vi "模态分析.vi"() -> ()   [LabVIEW 2014]
uses:
  <vilib>/Analysis/4window.llb/windowTd.ctl
  <vilib>/Utility/error.llb/DialogType.ctl
  <vilib>/Analysis/3filter.llb/Filter Structure Type.ctl
  <vilib>/DAQmx/read.llb/DAQmx Read (Analog 1D Wfm NChan NSamp).vi
  <vilib>/Analysis/2dsp.llb/Inverse Real FFT.vi
  <vilib>/DAQmx/create/channels.llb/DAQmx Create Channel (AI-Voltage-Basic).vi
  <vilib>/DAQmx/configure/timing.llb/DAQmx Timing (Sample Clock).vi
  <vilib>/DAQmx/miscellaneous.llb/DAQmx Fill In Error Info.vi
  <vilib>/measure/macond.llb/IIR Filter for 1 Chan.vi
  <vilib>/measure/maspectr.llb/Frequency Response Function (Mag-Phase) 1-1.vi
  <vilib>/measure/NI_MAPro.lvlib
  <vilib>/Analysis/NI_AALPro.lvlib
  <vilib>/Analysis/NI_AALBase.lvlib
panel:
  in  "units 2":i32(ring)=10348 caption="单位" items=["伏特"=10348, "来自自定义换算"=10065]
  in  "units":i32(ring)=10348 caption="单位" items=["伏特"=10348, "来自自定义换算"=10065]
  in  "触发阈值":dbl
  in  "Upper Fc":dbl
  in  "Lower Fc":dbl
  in  "Order":i32
  out "X":dbl[](array[numeric])
  in  "averaging mode":T1(ring)
  in  "是否转换成dB":bool=TRUE
  out "相关函数":cluster{"f0":dbl, "df":dbl, "coherence":dbl[]}(graph)
  out "相位":cluster{"f0":dbl, "df":dbl, "phase":dbl[]}(graph)
  out "幅度":cluster{"f0":dbl, "df":dbl, "magnitude":dbl[]}(graph)
  in  "FRF Mode":enum16{"H1", "H2", "H3"}(ring) caption="FRF模式"
  in  "window":T2=1 caption="窗" items=["矩形"=0, "Hanning"=1, "Hamming"=2, "Blackman-Harris"=3, "Exact Blackman"=4, "Blackman"=5, "Flat Top"=6, "4阶Blackman-Harris "=7, "7阶Blackman-Harris"=8, "Low Sidelobe"=9, "Blackman Nuttall"=11, "三角"=30, "Bartlett-Hanning"=31, "Bohman"=32, "Parzen"=33, "Welch"=34, "Kaiser"=60, "Dolph-Chebyshev"=61, "高斯"=62]
  out "响应信号":waveform(dbl)(graph)
  out "激振信号":waveform(dbl)(graph)
  in  "number of samples per channel 2":i32=-1 caption="每通道采样数"
  in  "sample mode 2":i32(ring)=10178 caption="采样模式" items=["有限采样"=10178, "连续采样"=10123, "硬件定时单点"=12522]
  in  "rate 2":dbl=1000.0 caption="速率" format="%0.2f"
  in  "input terminal configuration 3":i32(ring)=-1 caption="输入接线端配置" items=["默认"=-1, "RSE"=10083, "NRSE"=10078, "差分"=10106, "伪差分"=12529]
  in  "DAQmx物理通道 2":tag
  in  "input terminal configuration 2":i32(ring)=-1 caption="输入接线端配置" items=["默认"=-1, "RSE"=10083, "NRSE"=10078, "差分"=10106, "伪差分"=12529]
  in  "DAQmx物理通道":tag
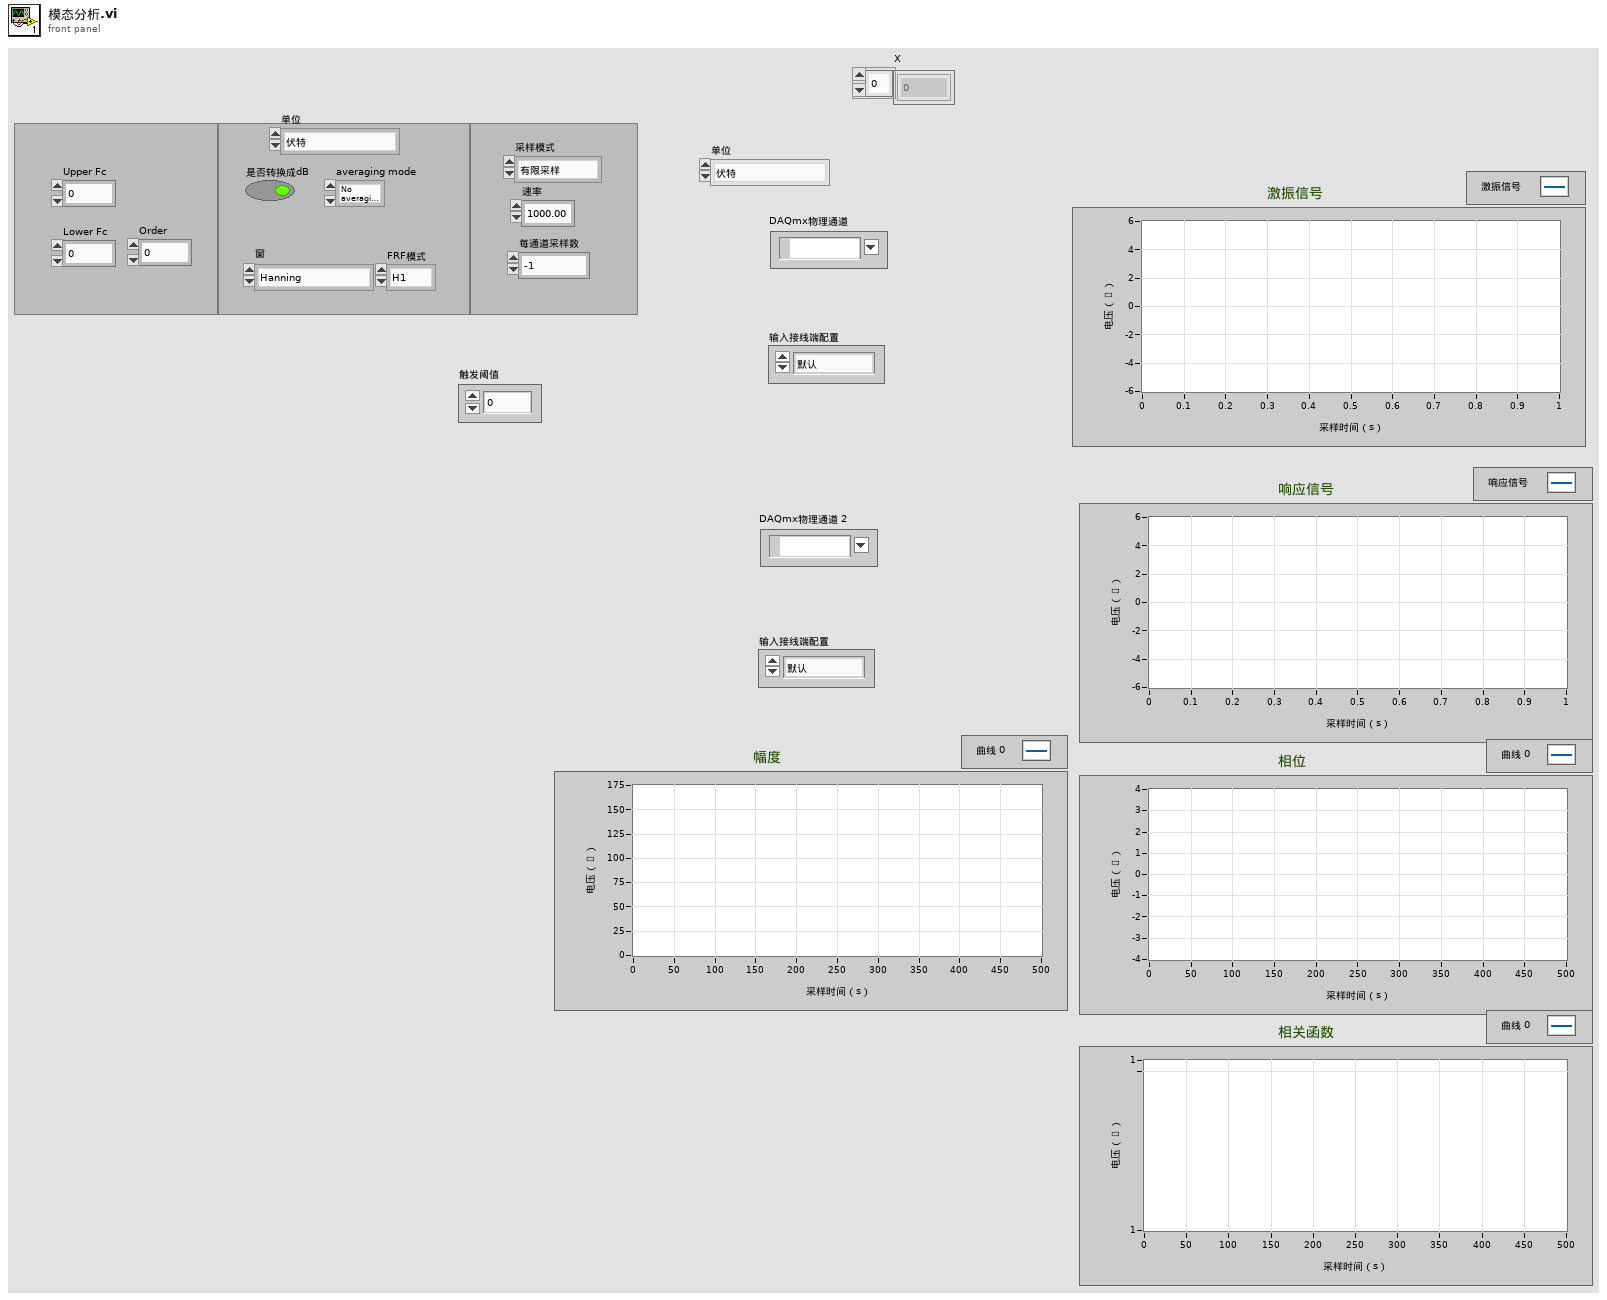
[diagram p1: front panel]
types:
  T1 = enum16{"No averaging", "Vector averaging", "RMS averaging", "Peak hold"}
  T2 = typedef "NI_AALPro.lvlib/windowTd.ctl" = u32
  T3 = typedef "NI_AALBase.lvlib/Filter Structure Type.ctl" = u16
  T4 = cluster{"Topology":enum16{"Off", "Butterworth", "Chebyshev", "Inverse Chebyshev", "Elliptic", "Bessel"}, "Type":enum16{"Lowpass", "Highpass", "Bandpass", "Bandstop"}, "Order":i32, "Lower Fc":dbl, "Upper Fc":dbl, "PB Ripple":dbl, "SB Attenuation":dbl}
  T5 = cluster{"averaging mode":enum16{"No averaging", "Vector averaging", "RMS averaging", "Peak hold"}, "weighting mode":enum16{"Linear", "Exponential"}, "number of averages":u32}
  T6 = cluster{"dB On (F)":bool, "unwrap phase (F)":bool, "convert to degree (F)":bool}
  T7 = typedef "DialogType.ctl" = u16
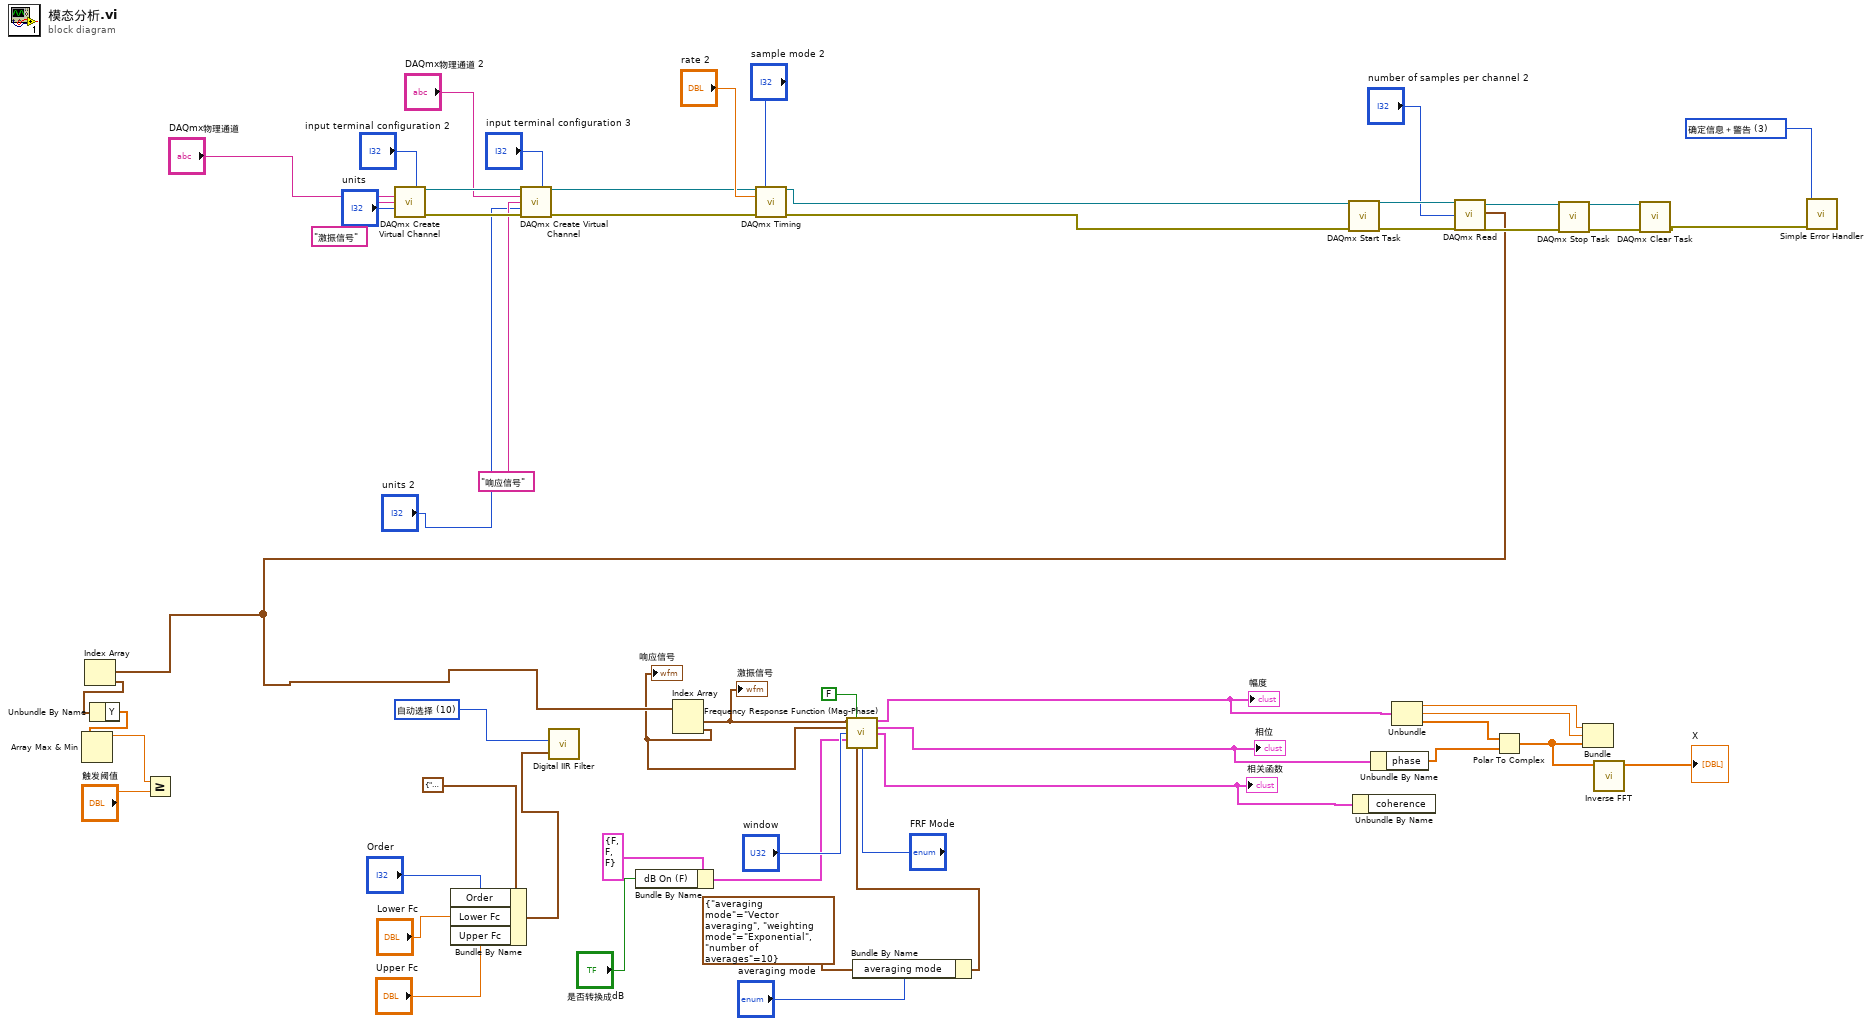
[diagram p0: block diagram]
diagram:
  w2 = T3 10 items=["IIR二阶"=0, "IIR四阶"=1, "自动选择"=10] ("filter structure option")
  w41 = T7 3 items=["无对话框", "确定信息", "继续或停止信息", "确定信息＋警告", "继续/停止+警告"] ("type of dialog (OK msg:1)")
  n1 = call-poly <vilib>:"DAQmx Create Virtual Channel.vi"("input terminal configuration"="input terminal configuration 2", "physical channels"="DAQmx物理通道", "name to assign"="激振信号", "units"="units") -> ("task out"=w53:refnum<k21>, "error out"=w52:errorcluster)  [unwired: 10 in]
  n2 = Bundle By Name(cluster=T4 {"Topology"=enum."Butterworth", "Type"=enum."Lowpass", "Order"=1, "Lower Fc"=100.0, "Upper Fc"=200.0, "PB Ripple"=1.0, "SB Attenuation"=60.0} ("IIR filter specifications"), "Order"="Order", "Lower Fc"="Lower Fc", "Upper Fc"="Upper Fc") -> (w14:T4)
  n3 = call-poly <vilib>:"DAQmx Create Virtual Channel.vi"("task in"=w53, "input terminal configuration"="input terminal configuration 3", "physical channels"="DAQmx物理通道 2", "name to assign"="响应信号", "units"="units 2", "error in"=w52) -> ("task out"=w37:refnum<k21>, "error out"=w36:errorcluster)  [unwired: 8 in]
  n4 = call-poly <vilib>:"Digital IIR Filter.vi"("IIR filter specifications"=w14, "filter structure option"=w2) -> ()  [unwired: 7 in, 3 out]
  n5 = Bundle By Name(cluster=T6 {"dB On (F)"=FALSE, "unwrap phase (F)"=FALSE, "convert to degree (F)"=FALSE} ("view"), "dB On (F)"="是否转换成dB") -> (w21:T6)
  n6 = call-poly <vilib>:"DAQmx Timing.vi"("task/channels in"=w37, "sample mode"="sample mode 2", "rate"="rate 2", "error in"=w36) -> ("task out"=w28:refnum<k21>, "error out"=w27:errorcluster)  [unwired: 10 in]
  n7 = Bundle By Name(cluster=T5 {"averaging mode"=enum."Vector averaging", "weighting mode"=enum."Exponential", "number of averages"=10} ("averaging parameters"), "averaging mode"="averaging mode") -> (w17:T5)
  n8 = call <vilib>:"DAQmx Start Task.vi"("task/channels in"=w28, "error in"=w27) -> ("task out"=w47:refnum<k21>, "error out"=w46:errorcluster)  [unwired: 12 in]
  n9 = call-poly <vilib>:"DAQmx Read.vi"("task/channels in"=w47, "number of samples per channel"="number of samples per channel 2", "error in"=w46) -> ("task out"=w45:refnum<k21>, "data"=w31:waveform(dbl)[], "error out"=w44:errorcluster)  [unwired: 10 in]
  n10 = Index Array(array=w31) -> (element=w35:waveform(dbl))  [unwired: 1 in]
  n11 = Unbundle By Name(w35) -> ("Y"=w34:dbl[])
  n12 = Array Max & Min(array=w34) -> (max value=w33:dbl)  [unwired: 3 out]
  n13 = Greater Or Equal?(x=w33, y="触发阈值") -> ()  [unwired: 1 out]
  n14 = Index Array(array=w31) -> (element #1=w4:waveform(dbl), element #2=w3:waveform(dbl))  [unwired: 2 in]
  "激振信号" <- w4
  "响应信号" <- w3
  n15 = call-poly <vilib>:"Frequency Response Function (Mag-Phase).vi"("time signal X"=w4, "restart averaging (F)"=FALSE, "time signal Y"=w3, "window"="window", "view"=w21, "averaging parameters"=w17, "FRF Mode"="FRF Mode") -> ("magnitude"=w26:cluster{"f0":dbl, "df":dbl, "magnitude":dbl[]}, "phase"=w25:cluster{"f0":dbl, "df":dbl, "phase":dbl[]}, "coherence"=w24:cluster{"f0":dbl, "df":dbl, "coherence":dbl[]})  [unwired: 3 in, 3 out]
  "幅度" <- w26
  "相位" <- w25
  "相关函数" <- w24
  n16 = Unbundle By Name(w24) -> ()  [unwired: 1 out]
  n17 = Unbundle By Name(w25) -> ("phase"=w9:dbl[])
  n18 = Unbundle(w26) -> ("f0"=w8:dbl, "df"=w7:dbl, "magnitude"=w10:dbl[])
  n19 = Polar To Complex(1:w9, 2:w10) -> (0:w6:cdb[])
  n20 = call <vilib>:"DAQmx Stop Task.vi"("task/channels in"=w45, "error in"=w44) -> ("task out"=w43:refnum<k21>, "error out"=w42:errorcluster)  [unwired: 12 in]
  n21 = Bundle("f0"=w8, "df"=w7, w6) -> ()  [unwired: 1 in, 1 out]
  n22 = call-poly <vilib>:"Inverse FFT.vi"("FFT {X}"=w6) -> ("X"=→"X":dbl[])  [unwired: 9 in, 1 out]
  n23 = call <vilib>:"DAQmx Clear Task.vi"("task in"=w43, "error in"=w42) -> ("error out"=w40:errorcluster)  [unwired: 13 in]
  n24 = call <vilib>:"Simple Error Handler.vi"("type of dialog (OK msg:1)"=w41, "error in (no error)"=w40) -> ()  [unwired: 3 in, 5 out]
